vi "Write T.vi"(8 "error in (no error)":errorcluster, 10 "t":T1, 11 "Domain_Evolut.lvclass in":refnum<class "NI_Domain_Evolut.lvclass">) -> (0 "error out":errorcluster, 3 "Domain_Evolut.lvclass out":refnum<class "NI_Domain_Evolut.lvclass">)   [LabVIEW 2017, in "NI_PDE.lvlib" / "NI_Domain_Evolut.lvclass"]
uses:
  <vilib>/gmath/pde.llb/DomainClass/Domain_Evolut/NI_Domain_Evolut.lvclass
  <vilib>/gmath/pde.llb/DomainClass/Domain_Evolut/NI_Domain_Evolut.lvclass/NI_Domain_Evolut.ctl
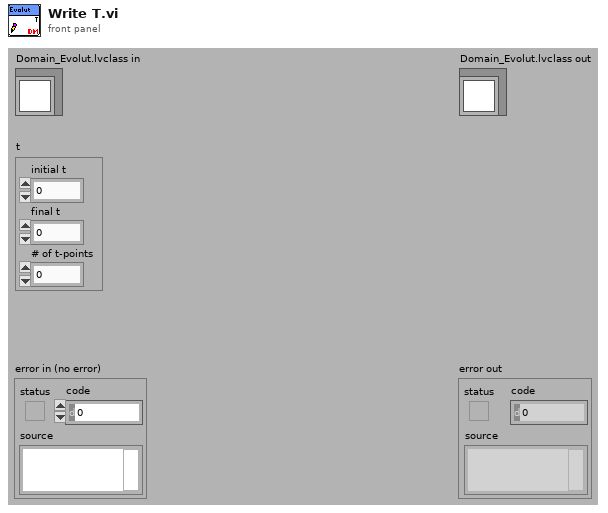
[diagram p1: front panel]
types:
  T1 = cluster{"initial t":dbl, "final t":dbl, "# of t-points":i32}
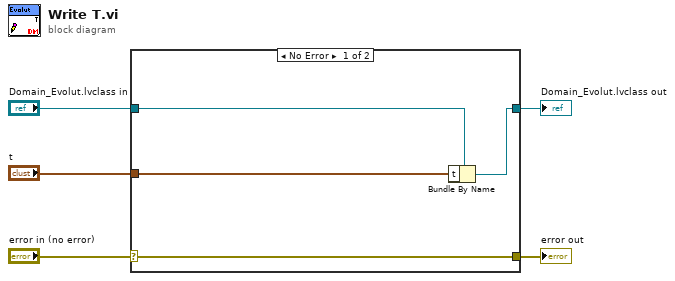
[diagram p0: block diagram]
diagram:
  n1 = case shown="No Error" "error in (no error)" {
    selector: "error in (no error)" -> [w9 w10]
    tunnel: [w9 w10] -> w4
    tunnel: [w7 w11] -> w2
    tunnel: "Domain_Evolut.lvclass in" -> [w8 w11]
    tunnel: "t" -> [w6 _]
    frame No Error {
      n2 = Bundle By Name(cluster=w8, "t"=w6) -> (w7:refnum<class "NI_Domain_Evolut.lvclass">)
    }
    frame Error {
    }
  }
  "error out" <- w4
  "Domain_Evolut.lvclass out" <- w2
